vi "Terminal-Test-Halt.vi"(8 "error in (no error)":errorcluster caption="错误输入（无错误）") -> (0 "error out":errorcluster caption="错误输出")   [LabVIEW 2014]
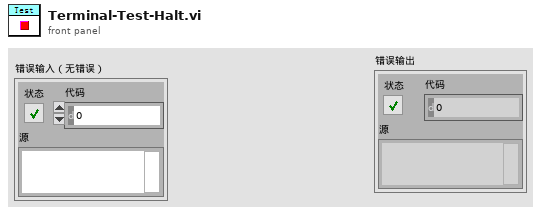
[diagram p1: front panel]
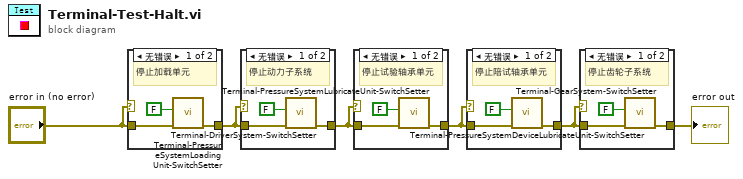
[diagram p0: block diagram]
diagram:
  n1 = case shown="无错误" "error in (no error)" {
    tunnel: "error in (no error)" -> [w9 w10]
    tunnel: [w7 w10] -> w4
    frame No Error {
      # "停止加载单元"
      n2 = call "Terminal-PressureSystemLoadingUnit-SwitchSetter.vi"("error in (no error)"=w9, "启停"=FALSE) -> ("error out"=w7:errorcluster)  [unwired: 9 in]
    }
    frame Error {
    }
  }
  n3 = case shown="无错误" w4 {
    tunnel: w4 -> [w12 w14]
    tunnel: [w11 w14] -> w3
    frame No Error {
      # "停止动力子系统"
      n4 = call "Terminal-DriverSystem-SwitchSetter.vi"("error in (no error)"=w12, "启停"=FALSE) -> ("error out"=w11:errorcluster)  [unwired: 9 in]
    }
    frame Error {
    }
  }
  n5 = case shown="无错误" w3 {
    tunnel: w3 -> [w16 w18]
    tunnel: [w15 w18] -> w2
    frame No Error {
      # "停止试验轴承单元"
      n6 = call "Terminal-PressureSystemLubricateUnit-SwitchSetter.vi"("error in (no error)"=w16, "启停"=FALSE) -> ("error out"=w15:errorcluster)  [unwired: 9 in]
    }
    frame Error {
    }
  }
  n7 = case shown="无错误" w2 {
    tunnel: w2 -> [w20 w22]
    tunnel: [w19 w22] -> w1
    frame No Error {
      # "停止陪试轴承单元"
      n8 = call "Terminal-PressureSystemDeviceLubricateUnit-SwitchSetter.vi"("error in (no error)"=w20, "启停"=FALSE) -> ("error out"=w19:errorcluster)  [unwired: 9 in]
    }
    frame Error {
    }
  }
  n9 = case shown="无错误" w1 {
    tunnel: w1 -> [w24 w26]
    tunnel: [w23 w26] -> w5
    frame No Error {
      # "停止齿轮子系统"
      n10 = call "Terminal-GearSystem-SwitchSetter.vi"("error in (no error)"=w24, "启停"=FALSE) -> ("error out"=w23:errorcluster)  [unwired: 9 in]
    }
    frame Error {
    }
  }
  "error out" <- w5
